vi "ModeDrivebase.vi"() -> (1 "Drive Mode Change":bool, 2 "Drive Mode":T1(ring))   [LabVIEW 2019]
doc: "This VI manages the robot drivebase mode. The default mode is driver control in which the swerve drive accepts all drive inputs and seemlessly combines them with autonomous heading corrections. Two auto targeting modes are also implimented."
uses:
  dscommands.vi
  sensors.vi
  dsdata.vi
  outputs.vi
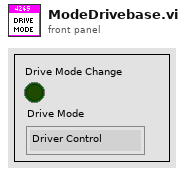
[diagram p1: front panel]
types:
  T1 = enum16{"Driver Control", "Auto Targeting", "Feeder Station"}
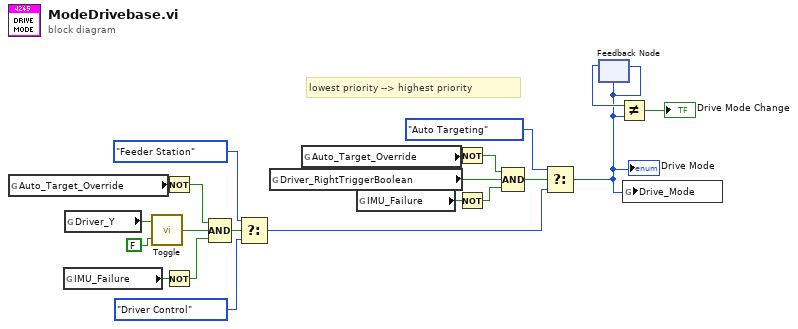
[diagram p0: block diagram]
diagram:
  # "lowest priority --> highest priority"
  n1 = global read "dsdata.vi" "Auto_Target_Override"() -> (w12:bool)
  n2 = global read "sensors.vi" "IMU_Failure"() -> (w10:bool)
  n3 = global read "dscommands.vi" "Driver_Y"() -> (w2:bool)
  n4 = call "Toggle.vi"("Initial State"=FALSE, "Trigger"=w2) -> ("New State"=w3:bool)
  n5 = Not(x=w12) -> (.not. x?=w11:bool)
  n6 = Not(x=w10) -> (.not. x?=w9:bool)
  n7 = Compound Arithmetic op=AND(w11, w3, w9) -> (w8:bool)
  n8 = Select(t=T1."Feeder Station", s=w8, f=T1."Driver Control") -> (s? t:f=w21:T1)
  n9 = global read "dscommands.vi" "Driver_RightTriggerBoolean"() -> (w19:bool)
  n10 = global read "dsdata.vi" "Auto_Target_Override"() -> (w18:bool)
  n11 = global read "sensors.vi" "IMU_Failure"() -> (w16:bool)
  n12 = Not(x=w18) -> (.not. x?=w17:bool)
  n13 = Not(x=w16) -> (.not. x?=w15:bool)
  n14 = Compound Arithmetic op=AND(w17, w19, w15) -> (w7:bool)
  n15 = Select(t=T1."Auto Targeting", s=w7, f=w21) -> (s? t:f=w4:T1)
  "Drive Mode" <- w4
  n16 = feedback #1(w4) -> (w6:T1)
  n17 = feedback-in #1(w4) -> ()
  n18 = Not Equal?(x=w6, y=w4) -> (x != y?=→"Drive Mode Change":bool)
  n19 = global write "outputs.vi" "Drive_Mode"(w4) -> ()
